vi "insert new and average.vi"(8 "Current step number":u32, 9 "Current loop number":u32, 10 "Current data array":dbl[](array[numeric]), 11 "Value to insert":dbl) -> (0 "Current step number":u32, 1 "Current loop number":u32, 2 "New data array":dbl[](array[numeric]))   [LabVIEW 2014]
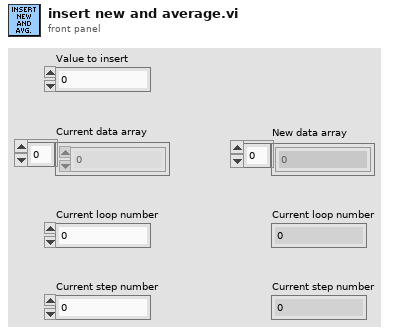
[diagram p1: front panel]
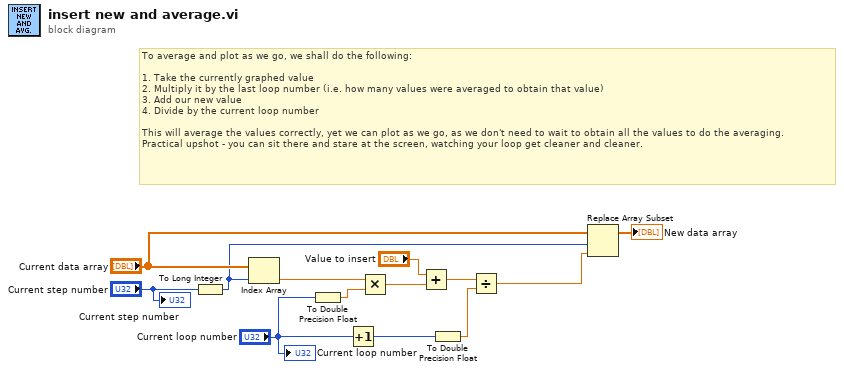
[diagram p0: block diagram]
diagram:
  # "To average and plot as we go, we shall do the following:\n\n1. Take the currently graphed value\n2. Multiply it by the last loop number (i.e. how many values were averaged to obtain that value)\n3. Add our new value\n4. Divide by the current loop number\n\nThis will average the values correctly, yet we can plot as we go, as we don't need to wait to obtain all the values to do the averaging.\nPractical upshot - you can sit there and stare at the screen, watching your loop get cleaner and cleaner."
  n1 = To Long Integer(number="Current step number") -> (32bit integer=w3:i32)
  n2 = Index Array(array="Current data array", index=w3) -> (element=w8:dbl)
  n3 = To Double Precision Float(number="Current loop number") -> (double precision float=w10:dbl)
  n4 = Increment(x="Current loop number") -> (x+1=w6:u32)
  n5 = Multiply(x=w8, y=w10) -> (x*y=w9:dbl)
  n6 = Add(x="Value to insert", y=w9) -> (x+y=w12:dbl)
  n7 = To Double Precision Float(number=w6) -> (double precision float=w11:dbl)
  n8 = Divide(x=w12, y=w11) -> (x/y=w2:dbl)
  n9 = Replace Array Subset(array="Current data array", new element=w2, index=w3) -> (→"New data array":dbl[])
  "Current loop number" <- "Current loop number"
  "Current step number" <- "Current step number"
